vi "ReportEnd_A170316-11.vi"(6 "文件重命名":bool, 8 "error in (no error)":errorcluster caption="错误输入（无错误）", 10 "文件名称":string, 11 "report in":refnum<class "NI_report.lvclass"> caption="报表输入") -> (0 "error out":errorcluster caption="错误输出")   [LabVIEW 2020]
uses:
  <vilib>/Utility/NIReport.llb/NI_report.lvclass
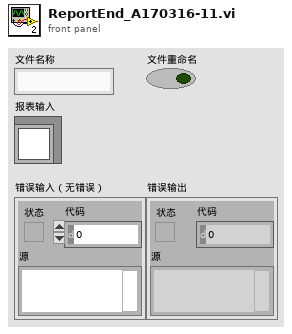
[diagram p1: front panel]
types:
  T1 = cluster{"Italic":enum16{"Italic Unchanged", "Italic On", "Italic Off"}, "Strike Through":enum16{"Strike Through Unchanged", "Strike Through On", "Strike Through Off"}, "Underline":enum16{"Underline Unchanged", "Underline On", "Underline Off"}, "Bold":enum16{"Bold Unchanged", "Bold On", "Bold Off"}}
  T2 = cluster{"Charset (-1)":i16, "Weight (-1)":i16, "Name":string, "Size":string}
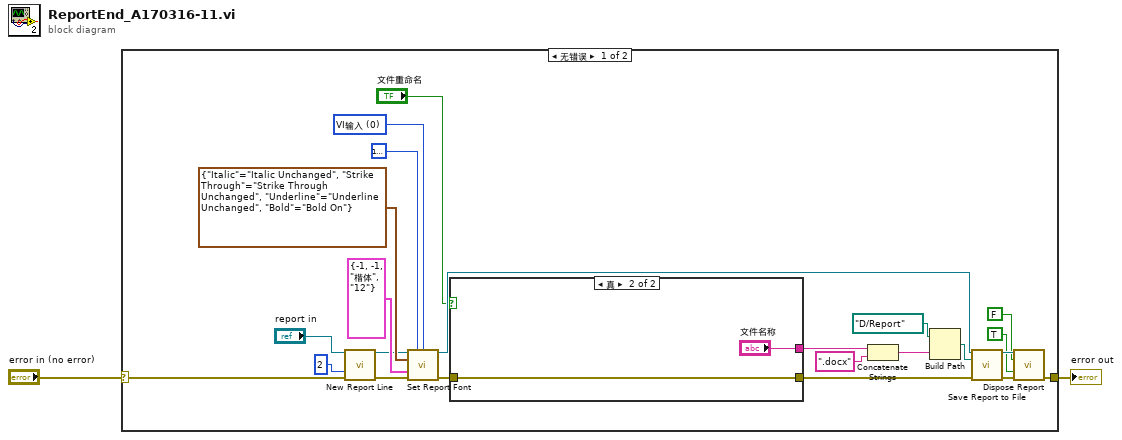
[diagram p0: block diagram]
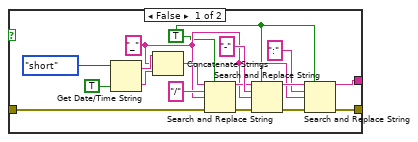
[diagram p2: hidden frame]
diagram:
  n1 = case shown="无错误" "error in (no error)" {
    selector: "error in (no error)" -> [w8 w45]
    tunnel: [w7 w45] -> w1
    frame No Error {
      w18 = u16 0 items=["VI输入", "字体对话框"] ("font settings source")
      n2 = call-dynamic "New Report Line.vi"("report in"="report in", "number of lines (1)"=2, "error in (no error)"=w8) -> ("report out"=w15:refnum<class "NI_report.lvclass">, "error out"=w14:errorcluster)  [unwired: 11 in]
      n3 = call-dynamic "Set Report Font.vi"("report in"=w15, "text color (unchanged)"=u32 16777224, "font settings source (VI Inputs)"=w18, "text options"=T1 {"Italic"=enum."Italic Unchanged", "Strike Through"=enum."Strike Through Unchanged", "Underline"=enum."Underline Unchanged", "Bold"=enum."Bold On"}, "font settings"=T2 {"Charset (-1)"=-1, "Weight (-1)"=-1, "Name"="楷体", "Size"="12"}, "error in (no error)"=w14) -> ("report out"=w11:refnum<class "NI_report.lvclass">, "error out"=w10:errorcluster)  [unwired: 7 in, 1 out]
      n4 = case shown="真" "文件重命名" {
        tunnel: [w37 "文件名称"] -> w5
        tunnel: w10 -> [w29 w43]
        tunnel: [w26 w43] -> w9
        frame False {
          w31 = TRUE ("替换全部？(F)")
          w32 = "_" ("替换字符串(\"\")")
          n5 = Get Date/Time String(date format (0)=enum16{"short", "long", "abbreviated"}."short" ("日期格式(0)"), want seconds? (F)=TRUE ("需要秒？(F)")) -> (date string=w42:string, time string=w38:string)  [unwired: 1 in]
          n6 = Concatenate Strings(w42, w32, w38) -> (w35:string)
          n7 = Search and Replace String(replace all?=w31, input string=w35, search string="/" ("搜索字符串"), replace string=w32, error in=w29) -> (result string=w34:string, error out=w28:errorcluster)  [unwired: 3 in, 2 out]
          n8 = Search and Replace String(replace all?=w31, input string=w34, search string="-" ("搜索字符串"), replace string=w32, error in=w28) -> (result string=w40:string, error out=w27:errorcluster)  [unwired: 3 in, 2 out]
          n9 = Search and Replace String(replace all?=w31, input string=w40, search string=":" ("搜索字符串"), replace string=w32, error in=w27) -> (result string=w37:string, error out=w26:errorcluster)  [unwired: 3 in, 2 out]
        }
        frame True {
        }
      }
      n10 = Concatenate Strings(w5, ".docx" ("字符串")) -> (w4:string)
      n11 = Build Path(base path=path "D:/Report" ("report file path"), name or relative path=w4) -> (appended path=w20:path)
      n12 = call-dynamic "Save Report to File.vi"("report in"=w11, "report file path"=w20, "error in (no error)"=w9) -> ("report out"=w25:refnum<class "NI_report.lvclass">, "error out"=w24:errorcluster)  [unwired: 11 in]
      n13 = call-dynamic "Dispose Report.vi"("report in"=w25, "wait until printing completed? (T)"=FALSE, "save changes? (F)"=TRUE, "error in (no error)"=w24) -> ("error out"=w7:errorcluster)  [unwired: 11 in]
    }
    frame Error {
    }
  }
  "error out" <- w1
